vi "PH_Cont-601k_PowerUnit.ProcState.vi"(0 "i ref in":refnum<vi>, 2 "state timeout":i32=-1, 4 "state":string, 5 "error in (no error)":errorcluster) -> (14 "i ref out":refnum<vi>, 18 "next state":string, 19 "error out":errorcluster)   [LabVIEW 2014, in "PH_Cont-601k_PowerUnit.lvlib"]
doc: "This VI represents part of the internal state machine of the object. All methods that are needed to implement the required functionality of the state machine will be called from THIS VI. Add your code here."
uses:
  PH_Cont-601k_PowerUnit.lvlib
  PH_Cont-601k_PSU/PH_Cont-601k_PSU.Configuration.ctl
  PH_PowerUnit_BaseClass/PH_PowerUnit_BaseClass.SM States.ctl
  PH_Cont-601k_PSU/PH_Cont-601k_PSU.Mode.ctl
  CSCore/CSSystem/CoreDefs/CoreDefs.error_type.ctl
  CSCore/CSSystem/CoreLib/CoreLib.lvlib
  CSCore/BaseSM/BaseSM.lvlib
  PH_PSDBWriter/PH_PSDBWriter.lvlib
  PH_PowerUnit_BaseClass/PH_PowerUnit_BaseClass.lvlib
  PH_Cont-601k_PSU/PH_Cont-601k_PSU.lvlib
  CSCore/CSSystem/CSSystemLib/CSSystemLib.lvlib
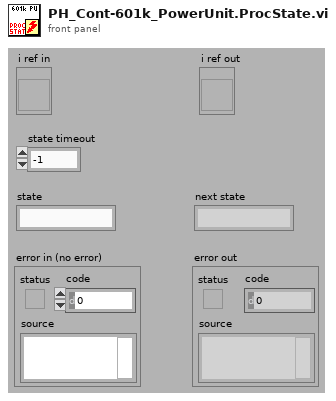
[diagram p1: front panel]
types:
  T1 = typedef "PH_PowerUnit_BaseClass.lvlib/PH_PowerUnit_BaseClass.SM States.ctl" = enum16{".", "Stand by", "Switch PU on", "Configure", "Set Default Voltage", "Set STANDBY", "Set READY", "Wait for Shot Cmd", "Open Dump Rods", "Open Ross Relais", "Close Ross Relais", "Switch PSU on", "Switch PSU off", "Charge", "Switch GD Channel on", "Close Dump Rods", "Rods-TO", "RR-TO", "PSU-TO", "Trigger-TO"}
  T2 = typedef "PH_Cont-601k_PSU.lvlib/PH_Cont-601k_PSU.Mode.ctl" = enum32{"STOP", "STANDBY", "READY", "EMISSION", "ERROR"}
  T3 = typedef "CoreDefs.error_type.ctl" = enum16{"no error", "can't load process", "can't unload process", "process does not exist", "can't install process", "can't remove process", "unknown function", "time out", "can't execute function", "duplicate queue name", "super not found", "caller queue invalid", "can't ping process", "unknown error", "VISA Error", "VISA timeout", "GPIB timeout", "GPIB error", "communication error", "data type mismatch", "can't read data from OPC server", "can't write data to OPC server", "OET error", "function not implemented", "process already exists", "invalid Shared Variable name", "error writing Shared Variable", "error reading Shared Variable", "invalid client name", "corrupt database", "unknown class", "call not authorized", "parameter out of range", "OET timeout: can't get data to modify", "invalid queue name", "requested operation incompatible with current state", "event undefined", "event disabled", "state undefined", "caller is not a friend", "EventBuilder: bad eventID", "EventBuilder: no DAQ devices", "a thread must not stop itself", "UNUSED ELEMENT4", "DiscArchiver: eventData incomplete", "DiscArchiver: eventData does not belong to run", "DiscArchiver: can't open file", "DiscArchiver: can't write to file", "DiscArchiver: available disc space low", "can't acquire semaphore", "error reading data from database", "notifier object is not existing", "can't register process", "can't unregister process", "illegal event type", "object disabled", "object already exists", "can't change state", "Instrument not found", "no connection to remote node", "invalid reference", "N/A", "UNUSED ELEMENT 1", "element not found", "illegal TCP/IP connection detected", "object does not exist", "invalid access ID", "unknown CS system", "invalid privilige", "unsupported data type", "unsupported server type", "IO server already exists", "Shared Variable already exists"}
  T4 = typedef "PH_PowerUnit_BaseClass.lvlib/PH_PowerUnit_BaseClass.i attribute.ctl" = cluster{"Constructor finished":bool, "PU":cluster{"In use":bool, "Service ID in use":i32, "GUI Ref":refnum<vi>}, "Enabling":cluster{"State":T5, "GUI Ref":refnum<vi>}, "Timing":cluster{"Last Shot":dbl, "Time between Shots [Sec]":dbl, "Waiting Time over?":bool, "Service ID Waiting Time":i32, "GUI Ref":refnum<vi>, "Instance":cluster{"Status":T6, "linked?":bool, "GUI Ref":refnum<vi>}}, "Sequencer":cluster{"SM State":string, "GUI Ref":refnum<vi>, "linked":bool}, "Subscribed Trendmssgs":cluster{"Tagname":string, "Status":T6, "linked?":bool, "Shot Condition":T6, "GUI Ref":refnum<vi>}[], "PP PU":T7, "Default Voltage (V)":dbl, "GUI Refs":T8, "PSDB data":cluster{"Shot Voltage [V]":dbl, "State TO SM":T1, "Write 2 early":bool}, "State TO SM":T1}
  T5 = typedef "PH_SystemInformation.lvlib/PH_SystemInformationEnabling State.ctl" = i32
  T6 = typedef "PH_StatusHandler.lvlib/PH_StatusHandler.Status.ctl" = i16
  T7 = typedef "PH_PP_Common.lvlib/PH_PP_Common.PUs.ctl" = enum16{"no Info", "PA-19mm-1", "PA-19mm-2", "PA-45mm-PILC", "PA-45mm-MAIN", "MA-PU-1", "MA-PU-2", "MA-PU-3", "MA-PU-4", "MA-PU-5", "MA-PU-6", "MA-FR", "MA-PILC", "PA-45mm-DP"}
  T8 = typedef "PH_PowerUnit_BaseClass.lvlib/PH_PowerUnit_BaseClass.GUI Refs.ctl" = cluster{"Delete Inst":refnum<vi>, "State TO SM":refnum<vi>, "State SM":refnum<vi>, "Fire":refnum<vi>}
  T9 = typedef "PH_Cont-601k_PSU.lvlib/PH_Cont-601k_PSU.Configuration.ctl" = u16
  T10 = typedef "PH_Cont-601k_PSU.lvlib/PH_Cont-601k_PSU.i attribute.ctl" = cluster{"GUI Refs":T11, "Interlock":bool, "Service ID applied Voltage":i32, "Device Settings":cluster{"Configuration":T9, "Flash Interval [s]":dbl, "Mode":T2, "Voltage [V]":u16, "Charge":bool, "VISA resource name":refnum<visa-resource-name>}, "Readyness":T12, "Information":cluster{"VISA resource name":refnum<visa-resource-name>, "Tagname Power On":string, "Interlock":cluster{"Instance":string, "Tagname":string}, "Limits [V]":cluster{"Lower":dbl, "Upper":dbl}, "Tagname PSU On":string}, "R2S":bool, "Charge is allowed":bool}
  T11 = typedef "PH_Cont-601k_PSU.lvlib/PH_Cont-601k_PSU.GUI Refs.ctl" = cluster{"Power On":refnum<vi>, "Hard- and Software":refnum<vi>, "Device Status":refnum<vi>, "Device Error":refnum<vi>, "Configuration":refnum<vi>, "Flash Interval [s]":refnum<vi>, "Interlock":refnum<vi>, "Interlock Indicator":refnum<vi>, "Voltage [V]":refnum<vi>, "Readyness":refnum<vi>, "Mode":refnum<vi>, "Reset Error":refnum<vi>, "Expert working":refnum<vi>, "Charge":refnum<vi>, "PSU On":refnum<vi>}
  T12 = typedef "PH_Cont-601k_PSU.lvlib/PH_Cont-601k_PSU.Readyness.ctl" = cluster{"Program":T13, "Device":T14}
  T13 = typedef "PH_Cont-601k_PSU.lvlib/PH_Cont-601k_PSU.Readyness Program.ctl" = enum32{"OFF", "POWER", "INTERLOCK"}
  T14 = typedef "PH_Cont-601k_PSU.lvlib/PH_Cont-601k_PSU.Readyness Device.ctl" = enum32{"OFF", "CONNECTING", "CONNECTED", "OPERATING", "EOC", "ERROR"}
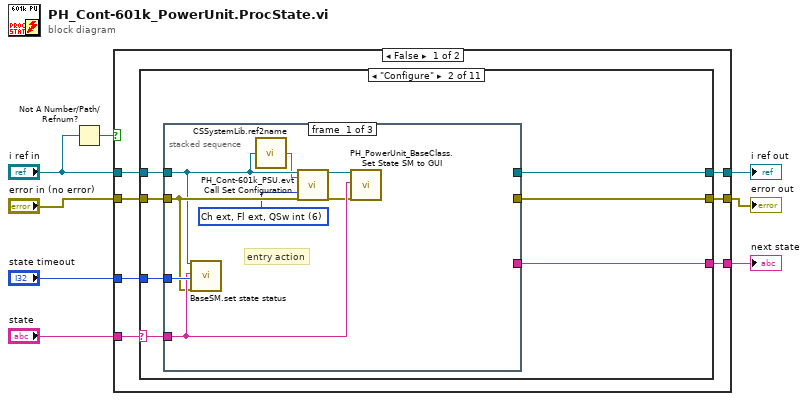
[diagram p0: block diagram]
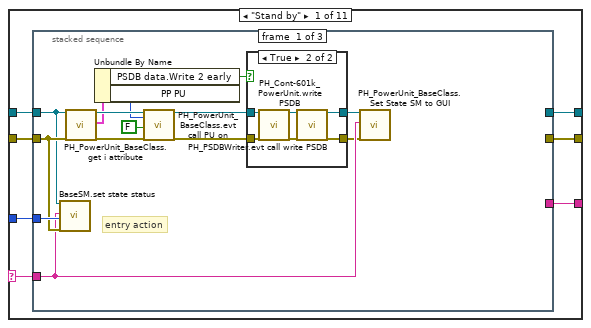
[diagram p2: hidden frame]
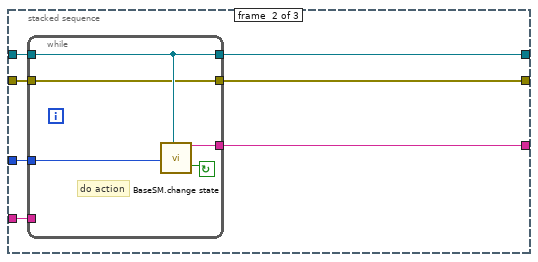
[diagram p4: hidden frame]
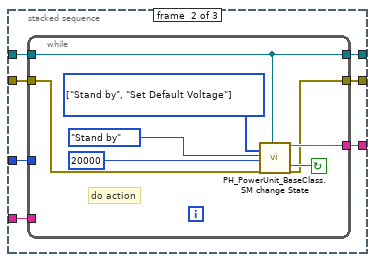
[diagram p6: hidden frame]
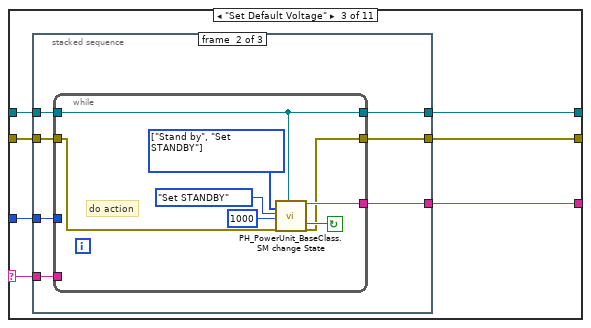
[diagram p8: hidden frame]
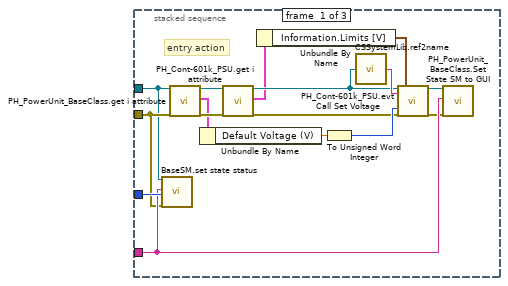
[diagram p9: hidden frame]
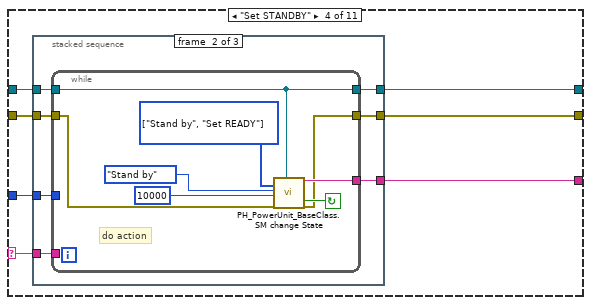
[diagram p11: hidden frame]
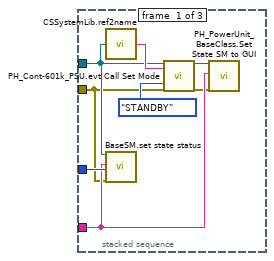
[diagram p12: hidden frame]
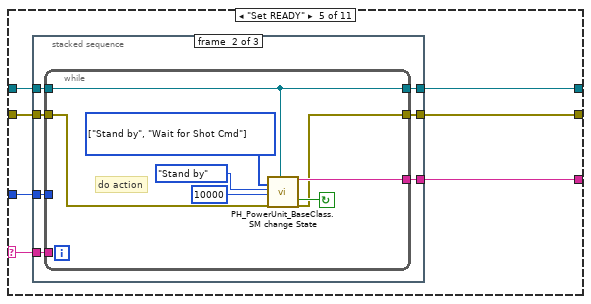
[diagram p14: hidden frame]
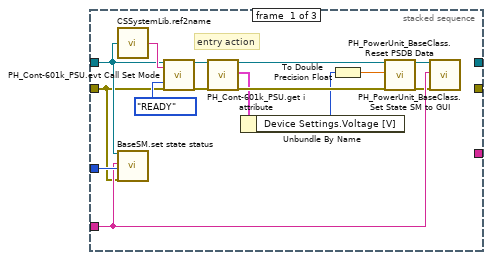
[diagram p15: hidden frame]
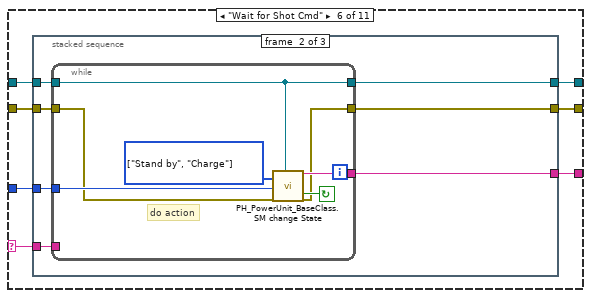
[diagram p17: hidden frame]
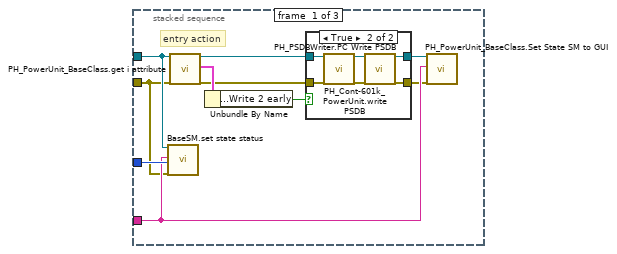
[diagram p18: hidden frame]
diagram:
  n1 = Not A Number/Path/Refnum?(number/path/refnum="i ref in") -> (NaN/Path/Refnum?=w2:bool)
  n2 = case shown="False" w2 {
    tunnel: "i ref in" -> [w15 w354]
    tunnel: [w14 w354] -> w8
    tunnel: "state" -> [w13 w351]
    tunnel: [w12 w351] -> w6
    tunnel: "state timeout" -> [w11 _]
    tunnel: "error in (no error)" -> [w10 _]
    tunnel: [w9 w352] -> w3
    frame False {
      n3 = case shown="\"Configure\"" w13 {
        selector: w13 -> [w22 w63 w93 w131 w161 w198 w237 w265 w296 w323 w345]
        tunnel: w15 -> [w20 w61 w91 w129 w159 w196 w235 w263 w294 w321 w350]
        tunnel: [w19 w60 w90 w128 w158 w195 w234 w262 w293 w320 w349] -> w14
        tunnel: [w21 w62 w92 w130 w160 w197 w236 w264 w295 w322 w344] -> w12
        tunnel: w11 -> [w18 w59 w89 w127 w157 w194 w233 w261 w292 w319 w346]
        tunnel: w10 -> [w17 w58 w88 w126 w156 w193 w232 w260 w291 w318 w348]
        tunnel: [w16 w57 w87 w125 w155 w192 w231 w259 w290 w317 w347] -> w9
        frame "Stand by" {
          n4 = stacked-sequence {
            tunnel: w22 -> [w34 w51 _]
            tunnel: [_ w50 _] -> w21
            tunnel: w20 -> [w31 w48 _]
            tunnel: [_ w47 _] -> w19
            tunnel: w18 -> [w36 w49 _]
            tunnel: w17 -> [w35 w45 _]
            tunnel: [_ w46 _] -> w16
            frame #0 {
              # "entry action"
              n5 = call "BaseSM.set state status.vi"("i ref in"=w31, "stateStatus"=w34, "ms timeout (10000)"=w36, "error in (no error)"=w35) -> ()  [unwired: 13 in, 3 out]
              n6 = call "PH_PowerUnit_BaseClass.get i attribute.vi"("i ref in"=w31, "error in (no error)"=w35) -> ("i ref out"=w30:refnum<vi>, "i attribute"=w29:T4, "error out"=w32:errorcluster)  [unwired: 15 in]
              n7 = Unbundle By Name(w29) -> ("PSDB data.Write 2 early"=w27:bool, "PP PU"=w28:T7)
              n8 = call "PH_PowerUnit_BaseClass.evt call PU on.vi"("i ref in"=w30, "PowerUnit"=w28, "PU on"=FALSE, "error in (no error)"=w32) -> ("i ref out"=w26:refnum<vi>, "error out"=w25:errorcluster)  [unwired: 14 in]
              n9 = case shown="True" w27 {
                tunnel: [w38 w40] -> w24
                tunnel: [w37 w39] -> w23
                tunnel: w26 -> [w38 w44]
                tunnel: w25 -> [w37 w43]
                frame False {
                }
                frame True {
                  n10 = call "PH_Cont-601k_PowerUnit.write PSDB.vi"("i ref in"=w44, "error IO"=w43) -> ("i ref out"=w41:refnum<vi>, "error out"=w42:errorcluster)  [unwired: 16 in]
                  n11 = call "PH_PSDBWriter.evt call write PSDB.vi"("i ref in"=w41, "error in (no error)"=w42) -> ("i ref out"=w40:refnum<vi>, "error out"=w39:errorcluster)  [unwired: 16 in]
                }
              }
              n12 = call "PH_PowerUnit_BaseClass.Set State SM to GUI.vi"("i ref in"=w24, "State SM"=w34, "error in (no error)"=w23) -> ()  [unwired: 15 in, 2 out]
            }
            frame #1 {
              n13 = while {
                tunnel: w49 -> [w54]
                tunnel: [w56] -> w50
                tunnel: w51 -> [_]
                tunnel: w48 -> [w53]
                tunnel: [w53] -> w47
                tunnel: [w52] -> w46
                tunnel: w45 -> [w52]
                stop <- w55 continue-if-true
                # "do action"
                n14 = call "BaseSM.change state.vi"("wait time [ms]"=w54, "i ref in"=w53) -> ("next state"=w56:string, "continue loop"=w55:bool)  [unwired: 14 in, 2 out]
              }
            }
            frame #2 {
              # "exit action"
            }
          }
        }
        frame "Configure" {
          n15 = stacked-sequence {
            tunnel: w63 -> [w70 w78 _]
            tunnel: [_ w77 _] -> w62
            tunnel: w61 -> [w65 w75 _]
            tunnel: [_ w74 _] -> w60
            tunnel: w59 -> [w71 w76 _]
            tunnel: w58 -> [w68 w72 _]
            tunnel: [_ w73 _] -> w57
            frame #0 {
              w66 = T9 6 items=["Ch intl, Fl intl, QSw intl", "Ch intl, Fl intl, QSw ext", "Ch intl, Fl ext, QSw intl", "Ch intl, Fl ext, QSw ext", "Ch ext, Fl int, QSw int", "Ch ext, Fl int, QSw ext", "Ch ext, Fl ext, QSw int", "Ch ext, Fl ext, QSw ext"] ("Configuration to set")
              # "entry action"
              n16 = call "BaseSM.set state status.vi"("i ref in"=w65, "stateStatus"=w70, "ms timeout (10000)"=w71, "error in (no error)"=w68) -> ()  [unwired: 13 in, 3 out]
              n17 = call "CSSystemLib.ref2name.vi"("obj refnum"=w65) -> ("name"=w64:string)
              n18 = call "PH_Cont-601k_PSU.evt Call Set Configuration.vi"("i ref in"=w65, "Instance name"=w64, "Configuration to set"=w66, "error in"=w68) -> ("i ref out"=w69:refnum<vi>, "error out"=w67:errorcluster)  [unwired: 14 in]
              n19 = call "PH_PowerUnit_BaseClass.Set State SM to GUI.vi"("i ref in"=w69, "State SM"=w70, "error in (no error)"=w67) -> ()  [unwired: 15 in, 2 out]
            }
            frame #1 {
              n20 = while {
                tunnel: w76 -> [_]
                tunnel: [w86] -> w77
                tunnel: w78 -> [_]
                tunnel: w75 -> [w84]
                tunnel: [w84] -> w74
                tunnel: [w81] -> w73
                tunnel: w72 -> [w82]
                stop <- w85 continue-if-true
                w79 = T1[] [enum."Stand by", enum."Set Default Voltage"] items=[".", "Stand by", "Switch PU on", "Configure", "Set Default Voltage", "Set STANDBY", "Set READY", "Wait for Shot Cmd", "Open Dump Rods", "Open Ross Relais", "Close Ross Relais", "Switch PSU on", "Switch PSU off", "Charge", "Switch GD Channel on", "Close Dump Rods", "Rods-TO", "RR-TO", "PSU-TO", "Trigger-TO"] ("allowed next states")
                # "do action"
                n21 = call "PH_PowerUnit_BaseClass.SM change State.vi"("allowed next states"=w79, "default state"=PH_PowerUnit_BaseClass.SM_States."Stand by", "wait time [ms]"=20000, "error in (no error)"=w82, "VI in"=w84) -> ("next state"=w86:string, "continue loop"=w85:bool, "error out"=w81:errorcluster)  [unwired: 12 in]
              }
            }
            frame #2 {
              # "exit action"
            }
          }
        }
        frame "Set Default Voltage" {
          n22 = stacked-sequence {
            tunnel: w93 -> [w108 w116 _]
            tunnel: [_ w115 _] -> w92
            tunnel: w91 -> [w102 w113 _]
            tunnel: [_ w112 _] -> w90
            tunnel: w89 -> [w109 w114 _]
            tunnel: w88 -> [w106 w110 _]
            tunnel: [_ w111 _] -> w87
            frame #0 {
              # "entry action"
              n23 = call "BaseSM.set state status.vi"("i ref in"=w102, "stateStatus"=w108, "ms timeout (10000)"=w109, "error in (no error)"=w106) -> ()  [unwired: 13 in, 3 out]
              n24 = call "PH_PowerUnit_BaseClass.get i attribute.vi"("i ref in"=w102, "error in (no error)"=w106) -> ("i ref out"=w97:refnum<vi>, "i attribute"=w101:T4, "error out"=w103:errorcluster)  [unwired: 15 in]
              n25 = Unbundle By Name(w101) -> ("Default Voltage (V)"=w100:dbl)
              n26 = call "PH_Cont-601k_PSU.get i attribute.vi"("i ref in"=w97, "error in (no error)"=w103) -> ("i ref out"=w96:refnum<vi>, "i attribute"=w95:T10, "error out"=w98:errorcluster)  [unwired: 15 in]
              n27 = Unbundle By Name(w95) -> ("Information.Limits [V]"=w94:cluster{"Lower":dbl, "Upper":dbl})
              n28 = To Unsigned Word Integer(number=w100) -> (unsigned 16bit integer=w99:u16)
              n29 = call "CSSystemLib.ref2name.vi"("obj refnum"=w96) -> ("name"=w104:string)
              n30 = call "PH_Cont-601k_PSU.evt Call Set Voltage.vi"("i ref in"=w96, "Instance name"=w104, "Voltage to set [V]"=w99, "error in"=w98, "Limits [V]"=w94) -> ("i ref out"=w107:refnum<vi>, "error out"=w105:errorcluster)  [unwired: 13 in]
              n31 = call "PH_PowerUnit_BaseClass.Set State SM to GUI.vi"("i ref in"=w107, "State SM"=w108, "error in (no error)"=w105) -> ()  [unwired: 15 in, 2 out]
            }
            frame #1 {
              n32 = while {
                tunnel: w114 -> [_]
                tunnel: [w124] -> w115
                tunnel: w116 -> [_]
                tunnel: w113 -> [w122]
                tunnel: [w122] -> w112
                tunnel: [w119] -> w111
                tunnel: w110 -> [w120]
                stop <- w123 continue-if-true
                w117 = T1[] [enum."Stand by", enum."Set STANDBY"] items=[".", "Stand by", "Switch PU on", "Configure", "Set Default Voltage", "Set STANDBY", "Set READY", "Wait for Shot Cmd", "Open Dump Rods", "Open Ross Relais", "Close Ross Relais", "Switch PSU on", "Switch PSU off", "Charge", "Switch GD Channel on", "Close Dump Rods", "Rods-TO", "RR-TO", "PSU-TO", "Trigger-TO"] ("allowed next states")
                # "do action"
                n33 = call "PH_PowerUnit_BaseClass.SM change State.vi"("allowed next states"=w117, "default state"=PH_PowerUnit_BaseClass.SM_States."Set STANDBY", "wait time [ms]"=1000, "error in (no error)"=w120, "VI in"=w122) -> ("next state"=w124:string, "continue loop"=w123:bool, "error out"=w119:errorcluster)  [unwired: 12 in]
              }
            }
            frame #2 {
              # "exit action"
            }
          }
        }
        frame "Set STANDBY" {
          n34 = stacked-sequence {
            tunnel: w131 -> [w138 w146 _]
            tunnel: [_ w145 _] -> w130
            tunnel: w129 -> [w133 w143 _]
            tunnel: [_ w142 _] -> w128
            tunnel: w127 -> [w139 w144 _]
            tunnel: w126 -> [w132 w140 _]
            tunnel: [_ w141 _] -> w125
            frame #0 {
              # "entry action"
              n35 = call "CSSystemLib.ref2name.vi"("obj refnum"=w133) -> ("name"=w135:string)
              n36 = call "BaseSM.set state status.vi"("i ref in"=w133, "stateStatus"=w138, "ms timeout (10000)"=w139, "error in (no error)"=w132) -> ()  [unwired: 13 in, 3 out]
              n37 = call "PH_Cont-601k_PSU.evt Call Set Mode.vi"("i ref in"=w133, "Instance name"=w135, "Mode to set"=PH_Cont-601k_PSU.Mode."STANDBY", "error in"=w132) -> ("i ref out"=w137:refnum<vi>, "error out"=w136:errorcluster)  [unwired: 14 in]
              n38 = call "PH_PowerUnit_BaseClass.Set State SM to GUI.vi"("i ref in"=w137, "State SM"=w138, "error in (no error)"=w136) -> ()  [unwired: 15 in, 2 out]
            }
            frame #1 {
              n39 = while {
                tunnel: w144 -> [_]
                tunnel: [w154] -> w145
                tunnel: w146 -> [_]
                tunnel: w143 -> [w152]
                tunnel: [w152] -> w142
                tunnel: [w149] -> w141
                tunnel: w140 -> [w150]
                stop <- w153 continue-if-true
                w147 = T1[] [enum."Stand by", enum."Set READY"] items=[".", "Stand by", "Switch PU on", "Configure", "Set Default Voltage", "Set STANDBY", "Set READY", "Wait for Shot Cmd", "Open Dump Rods", "Open Ross Relais", "Close Ross Relais", "Switch PSU on", "Switch PSU off", "Charge", "Switch GD Channel on", "Close Dump Rods", "Rods-TO", "RR-TO", "PSU-TO", "Trigger-TO"] ("allowed next states")
                # "do action"
                n40 = call "PH_PowerUnit_BaseClass.SM change State.vi"("allowed next states"=w147, "default state"=PH_PowerUnit_BaseClass.SM_States."Stand by", "wait time [ms]"=10000, "error in (no error)"=w150, "VI in"=w152) -> ("next state"=w154:string, "continue loop"=w153:bool, "error out"=w149:errorcluster)  [unwired: 12 in]
              }
            }
            frame #2 {
              # "exit action"
            }
          }
        }
        frame "Set READY" {
          n41 = stacked-sequence {
            tunnel: w161 -> [w175 w183 _]
            tunnel: [_ w182 _] -> w160
            tunnel: w159 -> [w172 w180 _]
            tunnel: [_ w179 _] -> w158
            tunnel: w157 -> [w176 w181 _]
            tunnel: w156 -> [w171 w177 _]
            tunnel: [_ w178 _] -> w155
            frame #0 {
              # "entry action"
              n42 = call "CSSystemLib.ref2name.vi"("obj refnum"=w172) -> ("name"=w174:string)
              n43 = call "BaseSM.set state status.vi"("i ref in"=w172, "stateStatus"=w175, "ms timeout (10000)"=w176, "error in (no error)"=w171) -> ()  [unwired: 13 in, 3 out]
              n44 = call "PH_Cont-601k_PSU.evt Call Set Mode.vi"("i ref in"=w172, "Instance name"=w174, "Mode to set"=PH_Cont-601k_PSU.Mode."READY", "error in"=w171) -> ("i ref out"=w166:refnum<vi>, "error out"=w169:errorcluster)  [unwired: 14 in]
              n45 = call "PH_Cont-601k_PSU.get i attribute.vi"("i ref in"=w166, "error in (no error)"=w169) -> ("i ref out"=w165:refnum<vi>, "i attribute"=w164:T10, "error out"=w167:errorcluster)  [unwired: 15 in]
              n46 = Unbundle By Name(w164) -> ("Device Settings.Voltage [V]"=w163:u16)
              n47 = To Double Precision Float(number=w163) -> (double precision float=w162:dbl)
              n48 = call "PH_PowerUnit_BaseClass.Reset PSDB Data.vi"("VI in"=w165, "PSDB data.Shot Voltage [V]"=w162, "error in (no error)"=w167) -> ("VI out"=w170:refnum<vi>, "error out"=w168:errorcluster)  [unwired: 15 in]
              n49 = call "PH_PowerUnit_BaseClass.Set State SM to GUI.vi"("i ref in"=w170, "State SM"=w175, "error in (no error)"=w168) -> ()  [unwired: 15 in, 2 out]
            }
            frame #1 {
              n50 = while {
                tunnel: w181 -> [_]
                tunnel: [w191] -> w182
                tunnel: w183 -> [_]
                tunnel: w180 -> [w189]
                tunnel: [w189] -> w179
                tunnel: [w186] -> w178
                tunnel: w177 -> [w187]
                stop <- w190 continue-if-true
                w184 = T1[] [enum."Stand by", enum."Wait for Shot Cmd"] items=[".", "Stand by", "Switch PU on", "Configure", "Set Default Voltage", "Set STANDBY", "Set READY", "Wait for Shot Cmd", "Open Dump Rods", "Open Ross Relais", "Close Ross Relais", "Switch PSU on", "Switch PSU off", "Charge", "Switch GD Channel on", "Close Dump Rods", "Rods-TO", "RR-TO", "PSU-TO", "Trigger-TO"] ("allowed next states")
                # "do action"
                n51 = call "PH_PowerUnit_BaseClass.SM change State.vi"("allowed next states"=w184, "default state"=PH_PowerUnit_BaseClass.SM_States."Stand by", "wait time [ms]"=10000, "error in (no error)"=w187, "VI in"=w189) -> ("next state"=w191:string, "continue loop"=w190:bool, "error out"=w186:errorcluster)  [unwired: 12 in]
              }
            }
            frame #2 {
              # "exit action"
            }
          }
        }
        frame "Wait for Shot Cmd" {
          n52 = stacked-sequence {
            tunnel: w198 -> [w207 w223 _]
            tunnel: [_ w222 _] -> w197
            tunnel: w196 -> [w202 w220 _]
            tunnel: [_ w219 _] -> w195
            tunnel: w194 -> [w208 w221 _]
            tunnel: w193 -> [w201 w217 _]
            tunnel: [_ w218 _] -> w192
            frame #0 {
              # "entry action"
              n53 = call "BaseSM.set state status.vi"("i ref in"=w202, "stateStatus"=w207, "ms timeout (10000)"=w208, "error in (no error)"=w201) -> ()  [unwired: 13 in, 3 out]
              n54 = call "PH_PowerUnit_BaseClass.get i attribute.vi"("i ref in"=w202, "error in (no error)"=w201) -> ("i ref out"=w205:refnum<vi>, "i attribute"=w206:T4, "error out"=w204:errorcluster)  [unwired: 15 in]
              n55 = Unbundle By Name(w206) -> ("PSDB data.Write 2 early"=w203:bool)
              n56 = case shown="True" w203 {
                tunnel: w205 -> [w210 w212]
                tunnel: w204 -> [w209 w211]
                tunnel: [w210 w214] -> w200
                tunnel: [w209 w213] -> w199
                frame False {
                }
                frame True {
                  n57 = call "PH_Cont-601k_PowerUnit.write PSDB.vi"("i ref in"=w212, "error IO"=w211) -> ("i ref out"=w215:refnum<vi>, "error out"=w216:errorcluster)  [unwired: 16 in]
                  n58 = call "PH_PSDBWriter.PC Write PSDB.vi"("i ref in"=w215, "error IO"=w216) -> ("i ref out"=w214:refnum<vi>, "error out"=w213:errorcluster)  [unwired: 16 in]
                }
              }
              n59 = call "PH_PowerUnit_BaseClass.Set State SM to GUI.vi"("i ref in"=w200, "State SM"=w207, "error in (no error)"=w199) -> ()  [unwired: 15 in, 2 out]
            }
            frame #1 {
              n60 = while {
                tunnel: w221 -> [w228]
                tunnel: [w230] -> w222
                tunnel: w223 -> [_]
                tunnel: w220 -> [w227]
                tunnel: [w227] -> w219
                tunnel: [w225] -> w218
                tunnel: w217 -> [w226]
                stop <- w229 continue-if-true
                w224 = T1[] [enum."Stand by", enum."Charge"] items=[".", "Stand by", "Switch PU on", "Configure", "Set Default Voltage", "Set STANDBY", "Set READY", "Wait for Shot Cmd", "Open Dump Rods", "Open Ross Relais", "Close Ross Relais", "Switch PSU on", "Switch PSU off", "Charge", "Switch GD Channel on", "Close Dump Rods", "Rods-TO", "RR-TO", "PSU-TO", "Trigger-TO"] ("allowed next states")
                # "do action"
                n61 = call "PH_PowerUnit_BaseClass.SM change State.vi"("allowed next states"=w224, "wait time [ms]"=w228, "error in (no error)"=w226, "VI in"=w227) -> ("next state"=w230:string, "continue loop"=w229:bool, "error out"=w225:errorcluster)  [unwired: 13 in]
              }
            }
            frame #2 {
              # "exit action"
            }
          }
        }
        frame "Charge" {
          n62 = stacked-sequence {
            tunnel: w237 -> [w243 w250 _]
            tunnel: [_ w249 _] -> w236
            tunnel: w235 -> [w241 w248 _]
            tunnel: [_ w247 _] -> w234
            tunnel: w233 -> [w244 _ _]
            tunnel: w232 -> [w242 w245 _]
            tunnel: [_ w246 _] -> w231
            frame #0 {
              # "entry action"
              n63 = call "BaseSM.set state status.vi"("i ref in"=w241, "stateStatus"=w243, "ms timeout (10000)"=w244, "error in (no error)"=w242) -> ()  [unwired: 13 in, 3 out]
              n64 = call "CSSystemLib.ref2name.vi"("obj refnum"=w241) -> ("name"=w240:string)
              n65 = call "PH_Cont-601k_PSU.evt Call Charge.vi"("i ref in"=w241, "Instance name"=w240, "error in"=w242) -> ("i ref out"=w239:refnum<vi>, "error out"=w238:errorcluster)  [unwired: 15 in]
              n66 = call "PH_PowerUnit_BaseClass.Set State SM to GUI.vi"("i ref in"=w239, "State SM"=w243, "error in (no error)"=w238) -> ()  [unwired: 15 in, 2 out]
            }
            frame #1 {
              n67 = while {
                tunnel: [w258] -> w249
                tunnel: w250 -> [_]
                tunnel: w248 -> [w256]
                tunnel: [w256] -> w247
                tunnel: [w253] -> w246
                tunnel: w245 -> [w254]
                stop <- w257 continue-if-true
                w251 = T1[] [enum."Stand by", enum."Switch GD Channel on", enum."PSU-TO"] items=[".", "Stand by", "Switch PU on", "Configure", "Set Default Voltage", "Set STANDBY", "Set READY", "Wait for Shot Cmd", "Open Dump Rods", "Open Ross Relais", "Close Ross Relais", "Switch PSU on", "Switch PSU off", "Charge", "Switch GD Channel on", "Close Dump Rods", "Rods-TO", "RR-TO", "PSU-TO", "Trigger-TO"] ("allowed next states")
                # "do action"
                n68 = call "PH_PowerUnit_BaseClass.SM change State.vi"("allowed next states"=w251, "default state"=PH_PowerUnit_BaseClass.SM_States."PSU-TO", "wait time [ms]"=20000 ("wait time"), "error in (no error)"=w254, "VI in"=w256) -> ("next state"=w258:string, "continue loop"=w257:bool, "error out"=w253:errorcluster)  [unwired: 12 in]
              }
            }
            frame #2 {
              # "exit action"
            }
          }
        }
        frame "Switch GD Channel on" {
          n69 = stacked-sequence {
            tunnel: w265 -> [w268 w275 _]
            tunnel: [_ w274 _] -> w264
            tunnel: w263 -> [w267 w273 w285]
            tunnel: [_ w272 _] -> w262
            tunnel: w261 -> [w269 _ _]
            tunnel: w260 -> [w266 w270 w284]
            tunnel: [_ w271 _] -> w259
            frame #0 {
              # "entry action"
              n70 = call "BaseSM.set state status.vi"("i ref in"=w267, "stateStatus"=w268, "ms timeout (10000)"=w269, "error in (no error)"=w266) -> ()  [unwired: 13 in, 3 out]
              n71 = call "PH_PowerUnit_BaseClass.Set State SM to GUI.vi"("i ref in"=w267, "State SM"=w268, "error in (no error)"=w266) -> ()  [unwired: 15 in, 2 out]
            }
            frame #1 {
              n72 = while {
                tunnel: [w283] -> w274
                tunnel: w275 -> [_]
                tunnel: w273 -> [w279]
                tunnel: [w279] -> w272
                tunnel: [w281] -> w271
                tunnel: w270 -> [w278]
                stop <- w282 continue-if-true
                w276 = T1[] [enum."Stand by", enum."Wait for Shot Cmd", enum."Trigger-TO"] items=[".", "Stand by", "Switch PU on", "Configure", "Set Default Voltage", "Set STANDBY", "Set READY", "Wait for Shot Cmd", "Open Dump Rods", "Open Ross Relais", "Close Ross Relais", "Switch PSU on", "Switch PSU off", "Charge", "Switch GD Channel on", "Close Dump Rods", "Rods-TO", "RR-TO", "PSU-TO", "Trigger-TO"] ("allowed next states")
                # "do action"
                n73 = call "PH_PowerUnit_BaseClass.SM change State.vi"("allowed next states"=w276, "default state"=PH_PowerUnit_BaseClass.SM_States."Trigger-TO", "wait time [ms]"=60000, "error in (no error)"=w278, "VI in"=w279) -> ("next state"=w283:string, "continue loop"=w282:bool, "error out"=w281:errorcluster)  [unwired: 12 in]
              }
            }
            frame #2 {
              # "exit action"
              n74 = Get Date/Time In Seconds() -> (seconds since 1Jan1904=w287:timestamp)
              n75 = To Double Precision Float(number=w287) -> (double precision float=w286:dbl)
              n76 = call "PH_Cont-601k_PowerUnit.update Last Shot Service.vi"("i ref in"=w285, "Last Shot"=w286, "error in (no error)"=w284) -> ("i ref out"=w288:refnum<vi>, "error out"=w289:errorcluster)  [unwired: 15 in]
              n77 = call "PH_PowerUnit_BaseClass.set Last Shot.vi"("VI in"=w288, "Last Shot"=w286, "error in (no error)"=w289) -> ()  [unwired: 15 in, 2 out]
            }
          }
        }
        frame "PSU-TO" {
          n78 = stacked-sequence {
            tunnel: w296 -> [w301 w308 _]
            tunnel: [_ w307 _] -> w295
            tunnel: w294 -> [w298 w306 _]
            tunnel: [_ w305 _] -> w293
            tunnel: w292 -> [w302 _ _]
            tunnel: w291 -> [w297 w303 _]
            tunnel: [_ w304 _] -> w290
            frame #0 {
              # "entry action"
              n79 = call "BaseSM.set state status.vi"("i ref in"=w298, "stateStatus"=w301, "ms timeout (10000)"=w302, "error in (no error)"=w297) -> ()  [unwired: 13 in, 3 out]
              n80 = call "PH_PowerUnit_BaseClass.handle TO.vi"("VI in"=w298, "String"=w301, "error in (no error)"=w297) -> ("VI out"=w300:refnum<vi>, "error out"=w299:errorcluster)  [unwired: 15 in]
              n81 = call "PH_PowerUnit_BaseClass.Set State SM to GUI.vi"("i ref in"=w300, "State SM"=w301, "error in (no error)"=w299) -> ()  [unwired: 15 in, 2 out]
            }
            frame #1 {
              n82 = while {
                tunnel: [w316] -> w307
                tunnel: w308 -> [_]
                tunnel: w306 -> [w314]
                tunnel: [w314] -> w305
                tunnel: [w312] -> w304
                tunnel: w303 -> [w313]
                stop <- w315 continue-if-true
                w309 = T1[] [enum."Stand by", enum."Switch PU on"] items=[".", "Stand by", "Switch PU on", "Configure", "Set Default Voltage", "Set STANDBY", "Set READY", "Wait for Shot Cmd", "Open Dump Rods", "Open Ross Relais", "Close Ross Relais", "Switch PSU on", "Switch PSU off", "Charge", "Switch GD Channel on", "Close Dump Rods", "Rods-TO", "RR-TO", "PSU-TO", "Trigger-TO"] ("allowed next states")
                # "do action"
                n83 = call "PH_PowerUnit_BaseClass.SM change State.vi"("allowed next states"=w309, "default state"=PH_PowerUnit_BaseClass.SM_States."Switch PU on", "wait time [ms]"=0 ("wait time"), "error in (no error)"=w313, "VI in"=w314) -> ("next state"=w316:string, "continue loop"=w315:bool, "error out"=w312:errorcluster)  [unwired: 12 in]
              }
            }
            frame #2 {
              # "exit action"
            }
          }
        }
        frame "Trigger-TO" {
          n84 = stacked-sequence {
            tunnel: w323 -> [w326 w335 _]
            tunnel: [_ w334 _] -> w322
            tunnel: w321 -> [w325 w333 _]
            tunnel: [_ w332 _] -> w320
            tunnel: w319 -> [w329 _ _]
            tunnel: w318 -> [w324 w330 _]
            tunnel: [_ w331 _] -> w317
            frame #0 {
              # "entry action"
              n85 = call "BaseSM.set state status.vi"("i ref in"=w325, "stateStatus"=w326, "ms timeout (10000)"=w329, "error in (no error)"=w324) -> ()  [unwired: 13 in, 3 out]
              n86 = call "PH_PowerUnit_BaseClass.handle TO.vi"("VI in"=w325, "String"=w326, "error in (no error)"=w324) -> ("VI out"=w328:refnum<vi>, "error out"=w327:errorcluster)  [unwired: 15 in]
              n87 = call "PH_PowerUnit_BaseClass.Set State SM to GUI.vi"("i ref in"=w328, "State SM"=w326, "error in (no error)"=w327) -> ()  [unwired: 15 in, 2 out]
            }
            frame #1 {
              n88 = while {
                tunnel: [w343] -> w334
                tunnel: w335 -> [_]
                tunnel: w333 -> [w341]
                tunnel: [w341] -> w332
                tunnel: [w339] -> w331
                tunnel: w330 -> [w340]
                stop <- w342 continue-if-true
                w337 = T1[] [enum."Stand by", enum."Switch PU on"] items=[".", "Stand by", "Switch PU on", "Configure", "Set Default Voltage", "Set STANDBY", "Set READY", "Wait for Shot Cmd", "Open Dump Rods", "Open Ross Relais", "Close Ross Relais", "Switch PSU on", "Switch PSU off", "Charge", "Switch GD Channel on", "Close Dump Rods", "Rods-TO", "RR-TO", "PSU-TO", "Trigger-TO"] ("allowed next states")
                # "do action"
                n89 = call "PH_PowerUnit_BaseClass.SM change State.vi"("allowed next states"=w337, "default state"=PH_PowerUnit_BaseClass.SM_States."Switch PU on", "wait time [ms]"=0 ("wait time"), "error in (no error)"=w340, "VI in"=w341) -> ("next state"=w343:string, "continue loop"=w342:bool, "error out"=w339:errorcluster)  [unwired: 12 in]
              }
            }
            frame #2 {
              # "exit action"
            }
          }
        }
        frame Default {
          n90 = call "BaseSM.ProcState.vi"("i ref in"=w350, "state timeout [ms]"=w346, "state"=w345, "error in (no error)"=w348) -> ("i ref out"=w349:refnum<vi>, "next state"=w344:string, "error out"=w347:errorcluster)  [unwired: 13 in]
        }
      }
    }
    frame True {
      n91 = call "CoreLib.my to LV error.vi"("ErrorTypes"=CoreDefs.error_type."invalid reference") -> ("myErrorCluster"=w352:errorcluster)  [unwired: 17 in, 1 out]
    }
  }
  "i ref out" <- w8
  "next state" <- w6
  "error out" <- w3
